vi "MF Send Task.vi"(8 "error in (no error)":errorcluster, 9 "Message Priority (Normal)":T2=enum."Normal", 10 "MsgType":cluster{"MF Msg Enum":T1, "Value":variant}, 11 "Message Enqueuer":refnum<class "Message Enqueuer.lvclass">) -> (0 "error out":errorcluster)   [LabVIEW 2024, in "MFActor.lvlib" / "MFActorMsg.lvclass"]
uses:
  MFActorMsg.lvclass
  <vilib>/ActorFramework/Message Enqueuer/Message Enqueuer.lvclass
  <vilib>/ActorFramework/Message Enqueuer/Message Priority.ctl
  MF Task Name.ctl
  C:/Program Files (x86)/National Instruments/LabVIEW 2024/vi.lib/ActorFramework/Message/Message.lvclass
  MFActorMsg.lvclass/MFActorMsg.ctl
  <vilib>/ActorFramework/Message Enqueuer/Message Enqueuer.lvclass/Message Enqueuer.ctl
  <vilib>/ActorFramework/Message Priority Queue/Priority Enqueue.vi
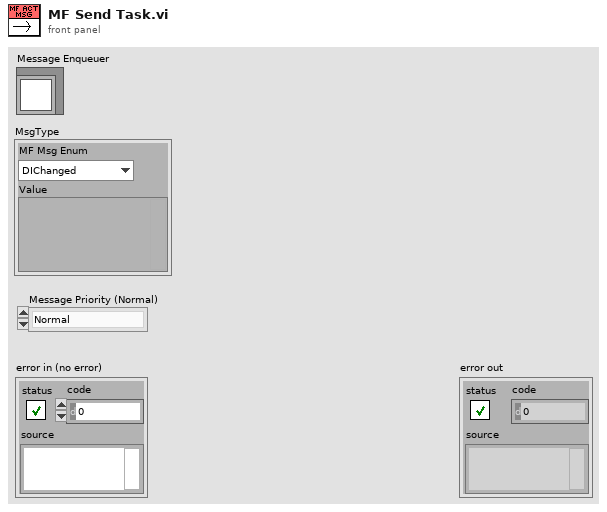
[diagram p1: front panel]
types:
  T1 = typedef "MF Task Name.ctl" = enum16{"DIChanged", "UpdateErrorCode", "SetTorque", "SetDriveTorque", "DataUpdated", "RunningTestProc", "StreamCtrl", "RunPID", "StopTest", "TCP Conn", "RefreshAutoUI", "ZeroAngle", "NestedActorLaunched", "NestedActorEnded", "ShowPsMsg"}
  T2 = typedef "Actor Framework.lvlib/Message Enqueuer.lvclass/Message Priority.ctl" = enum16{"Low", "Normal", "High"}
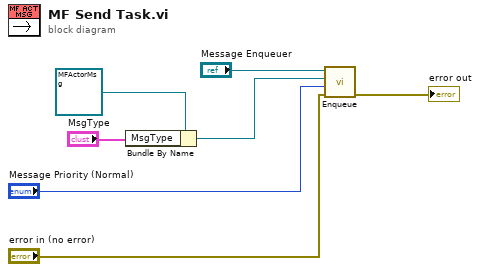
[diagram p0: block diagram]
diagram:
  n1 = Bundle By Name(cluster=refnum<class "MFActorMsg.lvclass"> refnum ("MFActor.lvlib:MFActorMsg.lvclass"), "MsgType"="MsgType") -> (w5:refnum<class "MFActorMsg.lvclass">)
  n2 = call <vilib>:"Enqueue.vi"("error in (no error)"="error in (no error)", "Message Priority (Normal)"="Message Priority (Normal)", "Message"=w5, "Message Enqueuer in"="Message Enqueuer") -> ("error out"=→"error out":errorcluster)  [unwired: 6 in, 1 out]
